vi "filewriter.vi"() -> ()   [LabVIEW 2020]
panel:
  in  "text":string
  in  "file path (use dialog)":path
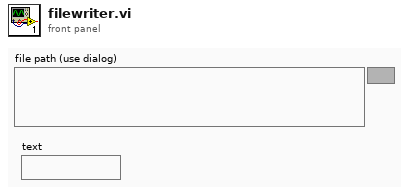
[diagram p1: front panel]
types:
  T1 = enum16{"open", "replace", "create", "open or create", "replace or create", "replace or create with confirmation"}
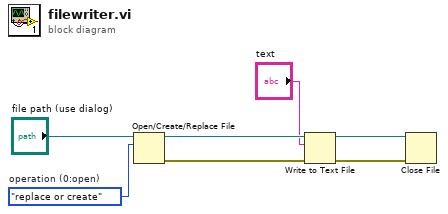
[diagram p0: block diagram]
diagram:
  w3 = T1."replace or create"  # operation (0:open)
  n1 = Open/Create/Replace File(file path (use dialog)="file path (use dialog)", operation (0:open)=w3) -> (refnum out=w7:refnum<file>, error out=w5:errorcluster)  [unwired: 4 in, 1 out]
  n2 = Write to Text File(file (use dialog)=w7, text="text", error in=w5) -> (refnum out=w6:refnum<file>, error out=w4:errorcluster)  [unwired: 1 in, 1 out]
  n3 = Close File(refnum=w6, error in=w4) -> ()  [unwired: 2 out]
